vi "HIOKI PW3390 Meas Harmonic.vi"(0 "VISA Resource":refnum<visa-resource-name>, 11 "error in (no error)":errorcluster, 13 "Error Out (F: Off)":bool) -> (3 "Status out":string, 4 "VISA Resource out":refnum<visa-resource-name>, 6 "Selected Item out":string[](array[string]), 8 "Data out":dbl[](array[numeric]), 10 "String out":string[](array[string]), 15 "error out":errorcluster)   [LabVIEW 2009]
doc: "Reads the Harmonic Measurement Data.\n\nReturns the measurement data specified by \"HIOKI PW3390 Conf Measure Item Harmonic.vi\". In this case, the measurement data's order is fixed. (Refer to output items and order)\n\nSelected Item out\n Returns the measurement item.\n\nData out\n Returns the measurement data.\nString out\n Returns the measurement data as string."
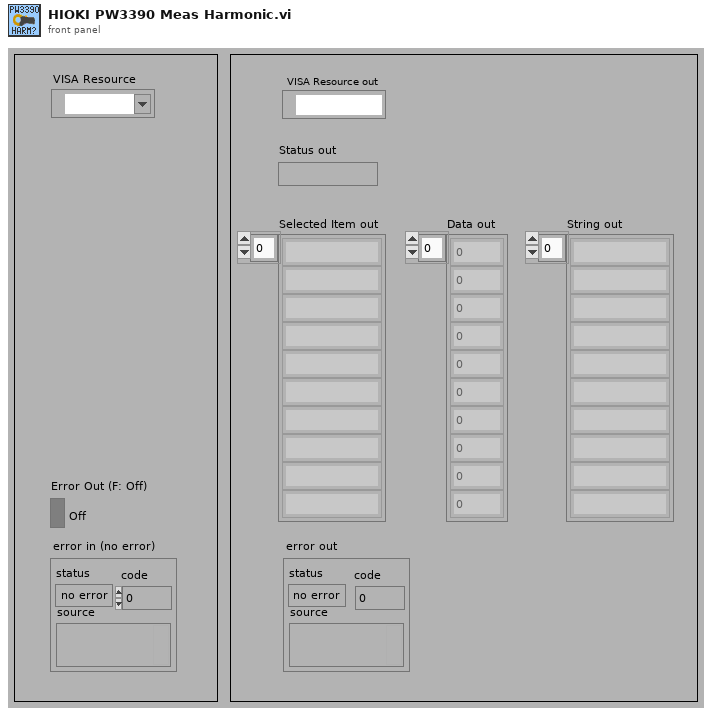
[diagram p1: front panel]
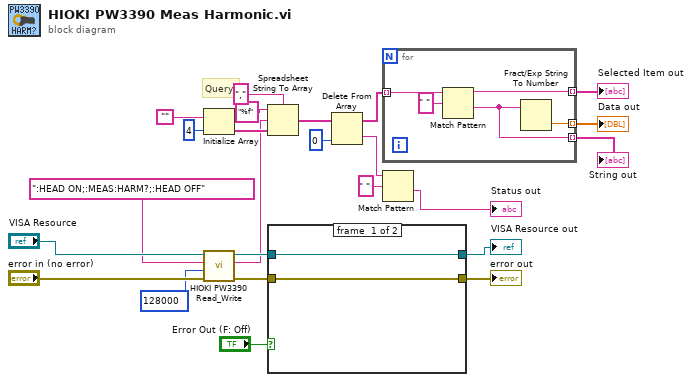
[diagram p0: block diagram]
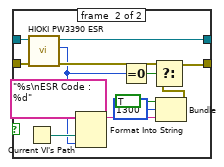
[diagram p2: hidden frame]
diagram:
  # "Query"
  n1 = Initialize Array("", 4) -> (w19:string[])
  n2 = call <instrlib>:"HIOKI PW3390 Read_Write.vi"("error in (no error)"="error in (no error)", "byte count (64000)"=u32 128000, "data in"=":HEAD ON;:MEAS:HARM?;:HEAD OFF", "VISA Resource"="VISA Resource") -> ("error out"=w22:errorcluster, "data out"=w14:string, "VISA Resource out"=w23:refnum<visa-resource-name>)  [unwired: 5 in]
  n3 = Spreadsheet String To Array(delimiter (Tab)=",", format string="%f", spreadsheet string=w14, array type (2D Dbl)=w19) -> (array=w11:string[])
  n4 = case shown="TRUE" "Error Out (F: Off)" {
    tunnel: w23 -> [w26 w39]
    tunnel: w22 -> [w25 w38]
    tunnel: [w25 w28] -> w21
    tunnel: [w26 w37] -> w9
    frame #0 {
    }
    frame #1 {
      n5 = Current VI's Path() -> (path=w35:path)
      n6 = call <instrlib>:"HIOKI PW3390 ESR.vi"("error in (no error)"=w38, "VISA Resource"=w39) -> ("error out"=w29:errorcluster, "Output Value"=w27:u8, "VISA Resource out"=w37:refnum<visa-resource-name>)  [unwired: 6 in, 1 out]
      n7 = Format Into String(format string="%s\nESR Code : %d", w35, w27) -> (resulting string=w31:string)  [unwired: 2 in, 1 out]
      n8 = Equal To 0?(x=w27) -> (x = 0?=w36:bool)
      n9 = Bundle("status"=TRUE, "code"=1300, w31) -> (w30:cluster{"status":bool, "code":i32, string})  [unwired: 1 in]
      n10 = Select(t=w29, s=w36, f=w30) -> (s? t:f=w28:errorcluster)
    }
  }
  "error out" <- w21
  "VISA Resource out" <- w9
  n11 = Delete From Array(array=w11, index=0 ("指標")) -> (deleted portion=w4:string, array with subset deleted=w8:string[])  [unwired: 1 in]
  n12 = for {
    tunnel: w8 -> [w44] mode=indexing
    tunnel: [w42] -> w5 mode=indexing
    tunnel: [w41] -> w6 mode=indexing
    tunnel: [w40] -> w7 mode=indexing
    n13 = Match Pattern(string=w44, regular expression=" ") -> (before substring=w40:string, after substring=w42:string)  [unwired: 1 in, 2 out]
    n14 = Fract/Exp String To Number(string=w42) -> (number=w41:dbl)  [unwired: 3 in, 1 out]
  }
  "Selected Item out" <- w7
  "Data out" <- w6
  "String out" <- w5
  n15 = Match Pattern(string=w4, regular expression=" ") -> (after substring=→"Status out":string)  [unwired: 1 in, 3 out]
